vi "Wait for Iteration Notification.vi"(8 "error in (no error)":errorcluster, 10 "timeout in ms (-1)":i32, 11 "Iterator NR Actor in":refnum<class "Iterator NR Actor.lvclass">) -> (0 "error out":errorcluster, 1 "timed out?":bool, 2 "Iterate?":bool, 3 "Iterator NR Actor out":refnum<class "Iterator NR Actor.lvclass">)   [LabVIEW 2023, in "Iterator Actor.lvlib" / "Iterator NR Actor.lvclass"]
uses:
  Iterator NR Actor.lvclass
  Iterator NR Actor.lvclass/Iterator NR Actor.ctl
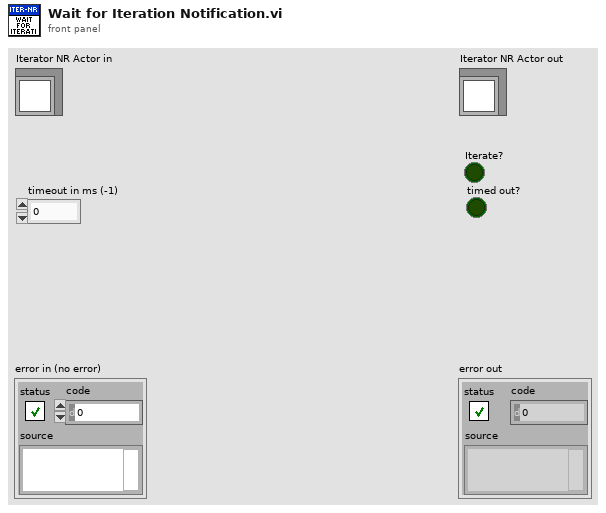
[diagram p1: front panel]
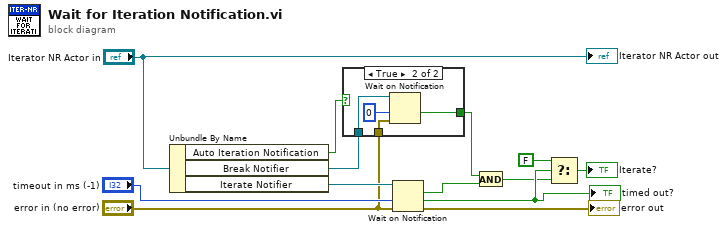
[diagram p0: block diagram]
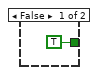
[diagram p2: hidden frame]
diagram:
  n1 = Unbundle By Name("Iterator NR Actor in") -> ("Auto Iteration Notification"=w4:bool, "Break Notifier"=w5:refnum<notifier>, "Iterate Notifier"=w12:refnum<notifier>)
  n2 = case shown="True" w4 {
    tunnel: "error in (no error)" -> [_ w18]
    tunnel: w5 -> [_ w17]
    tunnel: [TRUE ("timed out?") w15] -> w3
    frame False {
    }
    frame True {
      n3 = Wait on Notification(notifier=w17, timeout in ms (-1)=0, error in (no error)=w18) -> (timed out?=w15:bool)  [unwired: 1 in, 3 out]
    }
  }
  n4 = Wait on Notification(notifier=w12, timeout in ms (-1)="timeout in ms (-1)", error in (no error)="error in (no error)") -> (notification=w2:bool, timed out?=w9:bool, error out=→"error out":errorcluster)  [unwired: 1 in, 1 out]
  "timed out?" <- w9
  n5 = And(x=w3, y=w2) -> (x .and. y?=w1:bool)
  n6 = Select(t=FALSE, s=w9, f=w1) -> (s? t:f=→"Iterate?":bool)
  "Iterator NR Actor out" <- "Iterator NR Actor in"
